vi "generate.UUID.vi"() -> (3 "NI GUID":string)   [LabVIEW 2020]
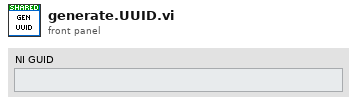
[diagram p1: front panel]
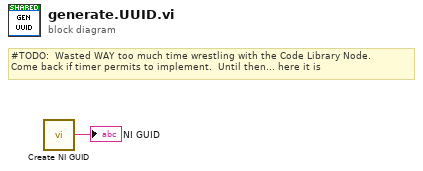
[diagram p0: block diagram]
diagram:
  # "#TODO:  Wasted WAY too much time wrestling with the Code Library Node.\nCome back if timer permits to implement.  Until then... here it is"
  n1 = call <vilib>:"Create NI GUID.vi"() -> ("NI GUID"=→"NI GUID":string)
